vi "SetProgramDataString.vi"(0 "VISA resource name":refnum<visa-resource-name>, 5 "get/set":T1, 7 "8800 Program Name (without .pgm extension)":string="test", 9 "Number of intervals in program":u16=1 min=1 max=300 step=1, 11 "error in (no error)":errorcluster) -> (4 "VISA resource name out":refnum<visa-resource-name>, 6 "8800 response":string, 15 "error out":errorcluster)   [LabVIEW 2023, in "Thermotron 8800.lvlib"]
doc: "PROG\nCommand name: Send or load program data string\nCommand type: Programming\nDescription: This command sets up the 8800 or host computer to load an entire program into the 8800’s program memory. The query command receives the data string from the 8800, while the operation command sends the data string to the 8800. For additional information, see “Using the interface command set” later in this section.\nThe query command sets up which program will be retrieved, and responds with the name of the program and the number of intervals in the program. The operation command sets up the name and the number of intervals in the program.\nSyntax: PROGname? or PROGn? or PROG, name, number of intervals\nWhere:\nname = program name\nnumber of intervals = integer (1 to 300)\nData type: See Syntax.\nQuery example: PROGtemp_test?\n8800 response: temp_test,6 (The program named “temp_test” is 6 intervals long.)\nOperation example: PROG,HI HUMIDITY,25\n8800 response: 0 (The 8800 will load a 25-interval program and name the program HI HUMIDITY.)"
uses:
  Thermotron 8800.lvlib
  Private/get set.ctl
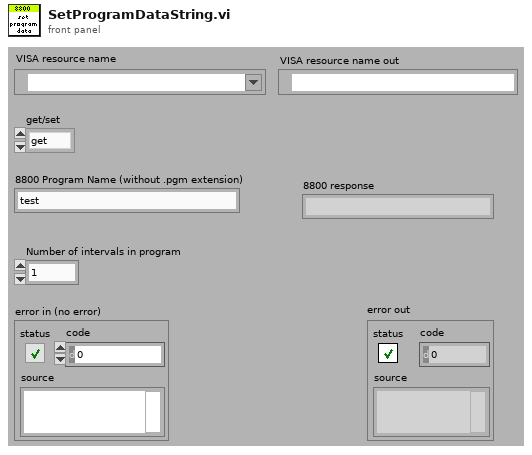
[diagram p1: front panel]
types:
  T1 = typedef "Thermotron 8800.lvlib/get set.ctl" = enum16{"get", "set"}
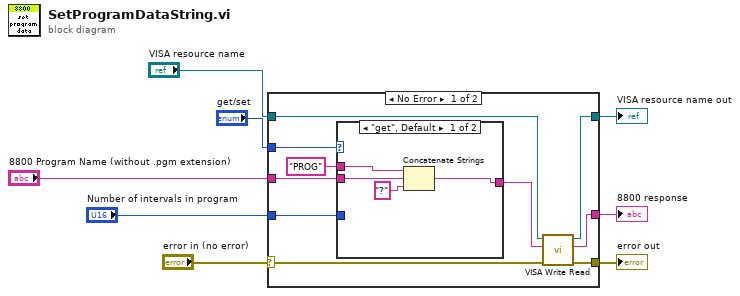
[diagram p0: block diagram]
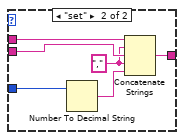
[diagram p2: hidden frame]
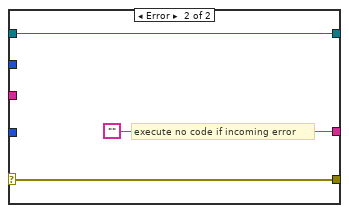
[diagram p3: hidden frame]
diagram:
  n1 = case shown="No Error" "error in (no error)" {
    selector: "error in (no error)" -> [w11 w31]
    tunnel: "VISA resource name" -> [w18 w30]
    tunnel: [w17 w30] -> w6
    tunnel: [w16 w31] -> w7
    tunnel: "8800 Program Name (without .pgm extension)" -> [w14 _]
    tunnel: "Number of intervals in program" -> [w13 _]
    tunnel: [w12 "" ("read buffer")] -> w3
    tunnel: "get/set" -> [w10 _]
    frame No Error {
      n2 = case shown="\"get\", Default" w10 {
        tunnel: "PROG" ("8800 Command") -> [w22 w28]
        tunnel: w14 -> [w21 w25]
        tunnel: w13 -> [_ w27]
        tunnel: [w19 w26] -> w9
        frame "get", Default {
          n3 = Concatenate Strings(w22, w21, "?" ("string")) -> (w19:string)
        }
        frame "set" {
          w24 = "," ("8800 Command")
          n4 = Number To Decimal String(number=w27) -> (decimal integer string=w23:string)  [unwired: 1 in]
          n5 = Concatenate Strings(w28, w24, w25, w24, w23) -> (w26:string)
        }
      }
      n6 = call "VISA Write Read.vi"("error in (no error)"=w11, "8800 Command"=w9, "VISA Refnum in"=w18) -> ("error out"=w16:errorcluster, "read buffer"=w12:string, "VISA Refnum out"=w17:refnum<visa-resource-name>)  [unwired: 6 in]
    }
    frame Error {
      # "execute no code if incoming error"
    }
  }
  "VISA resource name out" <- w6
  "error out" <- w7
  "8800 response" <- w3
